vi "stageGoRight.vi"() -> ()   [LabVIEW 2016]
uses:
  <vilib>/Instr/_visa.llb/VISA Configure Serial Port (Instr).vi
  variables/configDB.vi
panel:
  out "Moving":bool
  in  "Stage Position":string
  in  "Step length (um)":dbl=100.0
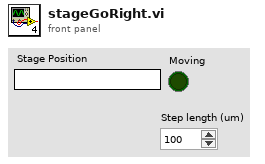
[diagram p1: front panel]
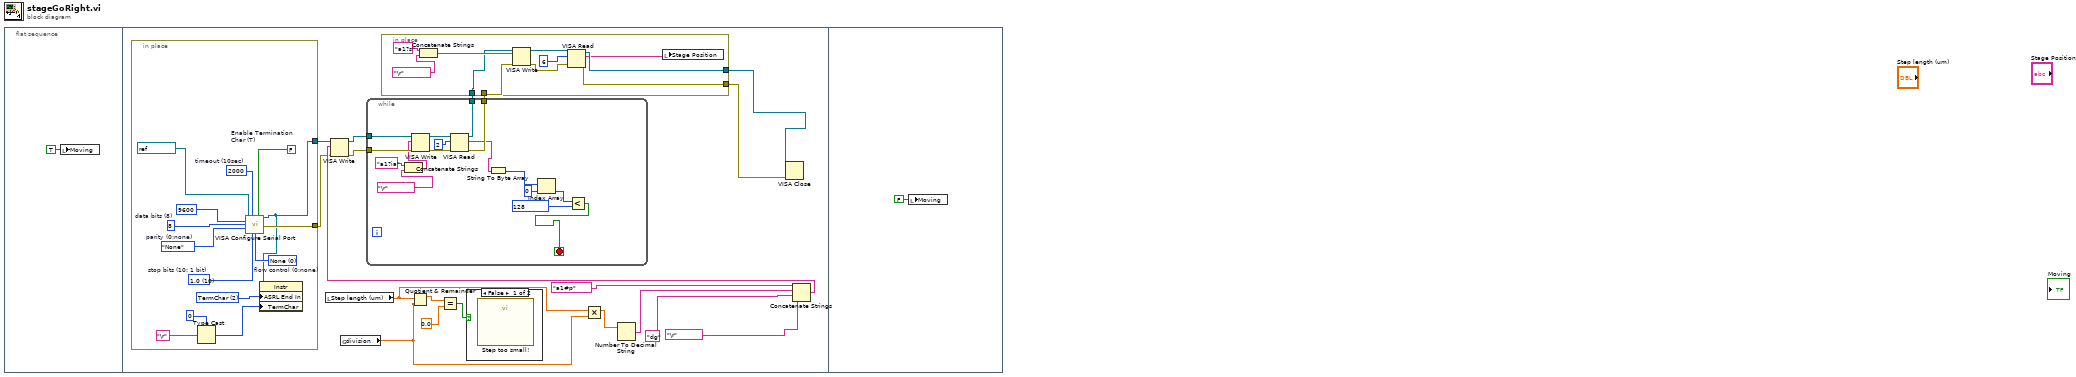
[diagram p0: block diagram]
diagram:
  n1 = flat-sequence {
    frame #0 {
      n2 = local write "Moving"(TRUE ("Moving")) -> ()
    }
    frame #1 {
      n3 = in-place {
        in-place-border: [w32] -> w15
        in-place-border: [w37] -> w14
        w33 = u16 2 items=["None", "Last Bit", "TermChar"] ("Serial Settings:End Mode for Reads")
        w39 = u16 0 items=["None", "XON/XOFF", "RTS/CTS", "XON/XOFF & RTS/CTS", "DTR/DSR", "XON/XOFF & DTR/DSR"]  # flow control (0:none)
        w40 = u16 10 items=["1.0"=10, "1.5"=15, "2.0"=20]  # stop bits (10: 1 bit)
        w41 = FALSE  # Enable Termination Char (T)
        w42 = u32 2000  # timeout (10sec)
        w43 = enum16{"None", "Odd", "Even", "Mark", "Space"}."None"  # parity (0:none)
        w44 = u16 8  # data bits (8)
        n4 = Type Cast(type=u8 0, x="\r") -> (*(type *) &x=w35:u8)
        n5 = call-poly "VISA Configure Serial Port"("VISA resource name"=refnum<visa-resource-name> "COM4", "timeout (10sec)"=w42, "Enable Termination\nChar (T)"=w41, "baud rate (9600)"=u32 9600, "data bits (8)"=w44, "parity (0:none)"=w43, "stop bits (10: 1 bit)"=w40, "flow control (0:none)"=w39) -> ("VISA resource name out"=w32:refnum<visa-resource-name>, "error out"=w37:errorcluster)  [unwired: 6 in]
        n6 = property class="Instr"(reference=w32, "ASRL End In"=w33, "TermChar"=w35) -> ()  [unwired: 1 in, 2 out]
      }
      n7 = local read "Step length (um)"() -> (w3:dbl)
      n8 = global read "configDB.vi" "division"() -> (w2:dbl)
      n9 = Quotient & Remainder(x=w3, y=w2) -> (x-y*floor(x/y)=w6:dbl)  [unwired: 1 out]
      n10 = Equal?(x=w6, y=0.0) -> (x = y?=w4:bool)
      n11 = case shown="False" w4 {
        frame False {
          n12 = call "Step too small!"() -> ()  [unwired: 18 in, 2 out]
        }
        frame True {
        }
      }
      n13 = Multiply(x=w3, y=w2) -> (x*y=w7:dbl)
      n14 = Number To Decimal String(number=w7) -> (decimal integer string=w19:string)  [unwired: 1 in]
      n15 = Concatenate Strings("a1#p" ("string"), w19, "dg" ("string"), "\r" ("write buffer")) -> (w20:string)
      n16 = VISA Write(VISA resource name=w15, write buffer=w20, error in (no error)=w14) -> (VISA resource name out=w13:refnum<visa-resource-name>, error out=w12:errorcluster)  [unwired: 1 out]
      n17 = while {
        tunnel: w13 -> [w61]
        tunnel: w12 -> [w60]
        tunnel: [w53] -> w11
        tunnel: [w52] -> w10
        stop <- w46 stop-if-true
        n18 = Concatenate Strings("a1?ia" ("write buffer"), "\r" ("write buffer")) -> (w57:string)
        n19 = VISA Write(VISA resource name=w61, write buffer=w57, error in (no error)=w60) -> (VISA resource name out=w56:refnum<visa-resource-name>, error out=w55:errorcluster)  [unwired: 1 out]
        n20 = VISA Read(VISA resource name=w56, byte count=u32 2, error in (no error)=w55) -> (VISA resource name out=w53:refnum<visa-resource-name>, read buffer=w51:string, error out=w52:errorcluster)  [unwired: 1 out]
        n21 = String To Byte Array(string=w51) -> (unsigned byte array=w50:u8[])
        n22 = Index Array(array=w50, index=0) -> (element=w48:u8)
        n23 = Less?(x=w48, y=u8 128) -> (x < y?=w46:bool)
      }
      n24 = in-place {
        in-place-border: w11 -> [w26]
        in-place-border: w10 -> [w25]
        in-place-border: [w24] -> w9
        in-place-border: [w23] -> w8
        n25 = Concatenate Strings("a1?s" ("write buffer"), "\r" ("write buffer")) -> (w29:string)
        n26 = VISA Write(VISA resource name=w26, write buffer=w29, error in (no error)=w25) -> (VISA resource name out=w30:refnum<visa-resource-name>, error out=w21:errorcluster)  [unwired: 1 out]
        n27 = VISA Read(VISA resource name=w30, byte count=u32 6, error in (no error)=w21) -> (VISA resource name out=w23:refnum<visa-resource-name>, read buffer=w22:string, error out=w24:errorcluster)  [unwired: 1 out]
        n28 = local write "Stage Position"(w22) -> ()
      }
      n29 = VISA Close(VISA resource name=w8, error in (no error)=w9) -> ()  [unwired: 1 out]
    }
    frame #2 {
      n30 = local write "Moving"(FALSE ("Moving")) -> ()
    }
  }
